vi "Control_DAQ_Loop.vi"(0 "DAQ":refnum<queue>, 2 "DAQ Control":T1, 11 "Error In":errorcluster) -> (15 "Error Out":errorcluster)   [LabVIEW 2023]
uses:
  type defs/DAQ_Control.ctl
  type defs/DAQ_States.ctl
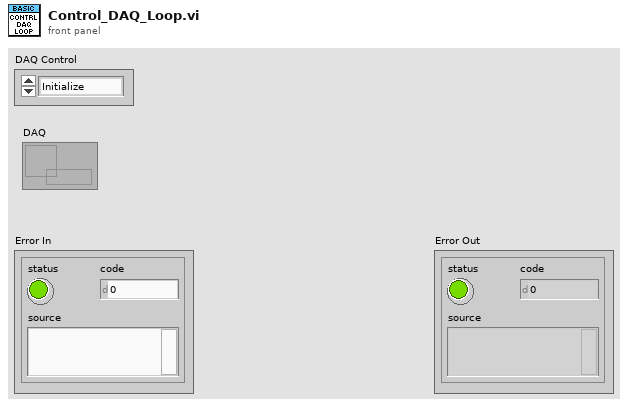
[diagram p1: front panel]
types:
  T1 = typedef "DAQ_Control.ctl" = enum16{"Initialize", "Shutdown", "Exit"}
  T2 = typedef "DAQ_States.ctl" = enum16{"Wait for Init", "Rename Devices", "Verify Hardware", "Initialize", "Run", "Shutdown", "Exit"}
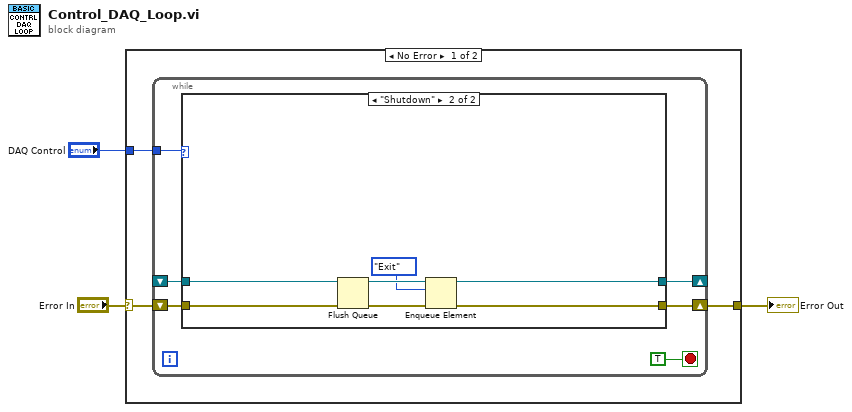
[diagram p0: block diagram]
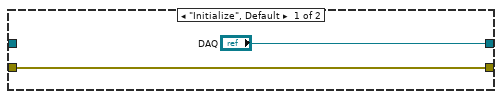
[diagram p2: hidden frame]
diagram:
  n1 = case shown="No Error" "Error In" {
    selector: "Error In" -> [w6 w22]
    tunnel: [w5 w22] -> w2
    tunnel: "DAQ Control" -> [w4 _]
    frame No Error {
      n2 = while {
        shift-right: [w10] -> w5
        shift-left: w6 -> [w11]
        shift-right: [w9] -> _
        shift-left: _ -> [w8]
        tunnel: w4 -> [w7]
        stop <- TRUE stop-if-true
        n3 = case shown="\"Shutdown\"" w7 {
          tunnel: w11 -> [w14 w21]
          tunnel: [w14 w18] -> w10
          tunnel: ["DAQ" w17] -> w9
          tunnel: w8 -> [_ w20]
          frame "Initialize", Default {
          }
          frame "Shutdown" {
            n4 = Flush Queue(queue=w20, error in (no error)=w21) -> (queue out=w16:refnum<queue>, error out=w19:errorcluster)  [unwired: 1 out]
            n5 = Enqueue Element(queue=w16, element=DAQ_States."Exit", error in (no error)=w19) -> (queue out=w17:refnum<queue>, error out=w18:errorcluster)  [unwired: 1 in, 1 out]
          }
        }
      }
    }
    frame Error {
    }
  }
  "Error Out" <- w2
